vi "Digital Pattern Gen Run Test.vi"() -> ()   [LabVIEW 2013]
uses:
  IP Source/APU/Settings.ctl
  IP Source/Digital Pattern Generation/Settings.ctl
  IP Source/APU/Input.ctl
  IP Source/Digital Pattern Generation/Load Input.ctl
  <vilib>/rvi/interface/RandomDataEmulation/nirviRandomDataOpen.vi
  <vilib>/rvi/interface/common/niFpgaCacheSessionInfoDynamic.vi
  <vilib>/rvi/interface/common/niFpgaWaitOnOcc.vi
  <vilib>/Utility/error.llb/Error Cluster From Error Code.vi
  <vilib>/rvi/errors/niLvFpgaAdjustHostInterfaceError.vi
  <vilib>/FPGAPlugInAG/Dynamic/niLvFpga_Run_Dynamic.vi
  <vilib>/FPGAPlugInAG/Dynamic/niLvFpga_Close_Dynamic.vi
  <vilib>/rvi/interface/nirviOpenFPGA/nirviOpenFPGA.xnode
  Compile Tests/APU + 4 Digital Patterns.vi
  <vilib>/rvi/interface/nirviReadWriteControl/nirviReadWriteControl.xnode
  <vilib>/rvi/interface/nirviMethod/nirviMethod.xnode
  <vilib>/rvi/interface/nirviCloseFPGA/nirviCloseFPGA.xnode
  <vilib>/rvi/interface/Simulation/niFpgaSimulationCallBeginRW.vi
  IP Source/APU/APU.lvlib
  IP Source/Digital Pattern Generation/Digital Pattern Generation.lvlib
  NiFpgaLv.dll
panel:
  in  "use fault count":bool
  in  "fault count":fxp<+,4,4>
  in  "fault value":bool
  in  "fault wrap":bool
  in  "fault":bool
  in  "edge 2":u16
  in  "edge 1":u16
  in  "slow load":bool=TRUE
  in  "cycle angle":bool
  in  "Tooth Angles":cluster{"Rising Edge":dbl, "Falling Edge":dbl}[](array[cluster])=[{"Rising Edge"=50.0, "Falling Edge"=60.0}, {"Rising Edge"=100.0, "Falling Edge"=110.0}, {"Rising Edge"=200.0, "Falling Edge"=300.0}]
  out "Load done":bool
  out "Load time (s)":dbl
  in  "RPM":dbl=100000.0 format="%#_15g"
  in  "stop":bool
  # "for simulation"
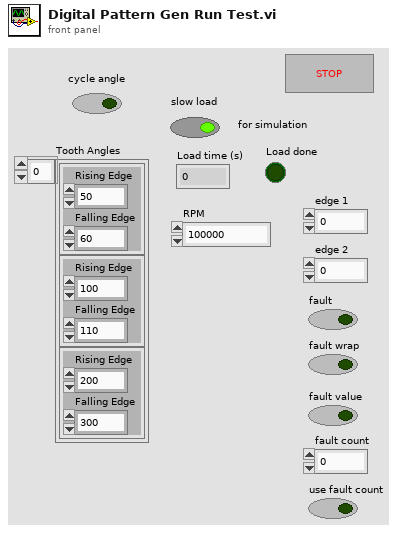
[diagram p1: front panel]
types:
  T1 = typedef "Engine Simulation Toolkit.lvlib/Digital Pattern Generation.lvlib/Settings.ctl" = cluster{"edge 1":u16, "edge 2":u16, "cycle angle":bool, "enabled":bool, "first falling":bool, "fault":bool, "fault wrap":bool, "fault value":bool, "fault count":fxp<+,4,4>, "use fault count":bool}
  T2 = typedef "Engine Simulation Toolkit.lvlib/APU.lvlib/Settings.ctl" = cluster{"acceleration":fxp<+,18,-20>, "enable accel":bool}
  T3 = typedef "Engine Simulation Toolkit.lvlib/Digital Pattern Generation.lvlib/Load Input.ctl" = cluster{"address":fxp<+,11,11>, "done":bool, "angle":u16}
  T4 = typedef "Engine Simulation Toolkit.lvlib/APU.lvlib/Input.ctl" = cluster{"desired speed":fxp<+/-,23,2>, "reset":bool}
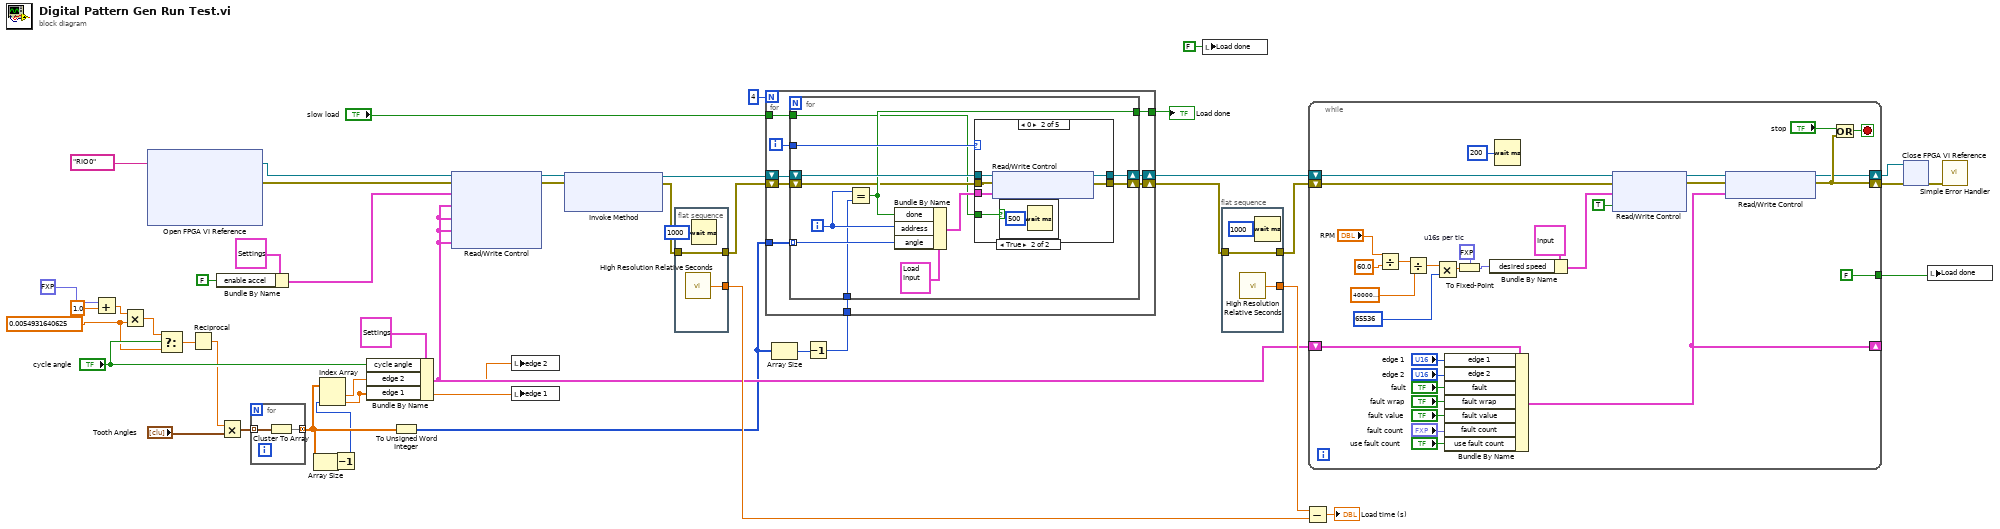
[diagram p0: block diagram]
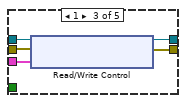
[diagram p4: hidden frame]
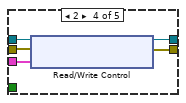
[diagram p5: hidden frame]
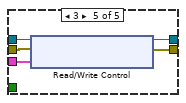
[diagram p6: hidden frame]
diagram:
  w18 = 0.0054931640625 ("x")
  n1 = Add(x=fxp<+,2,2> 1.0 ("extra cranks for a cycle"), y=1.0) -> (x+y=w6:dbl)
  n2 = Multiply(x=w6, y=w18) -> (x*y=w19:dbl)
  n3 = xnode "Open FPGA VI Reference"("resource name"=tag "RIO0") -> ("FPGA VI Reference Out"=w11:refnum<k20>, "error out"=w42:errorcluster)  [unwired: 1 in]
  n4 = Select(t=w19, s="cycle angle", f=w18) -> (s? t:f=w7:dbl)
  n5 = Reciprocal(x=w7) -> (1/x=w9:dbl)
  n6 = Bundle By Name(cluster=T2 {"acceleration"=0.0, "enable accel"=FALSE} ("settings with acceleration"), "enable accel"=FALSE) -> (w23:T2)
  n7 = Multiply(x=w9, y="Tooth Angles") -> (x*y=w16:cluster{"Rising Edge":dbl, "Falling Edge":dbl}[])
  n8 = for {
    tunnel: w16 -> [w47] mode=indexing
    tunnel: [w46] -> w14 mode=concatenating
    n9 = Cluster To Array(cluster=w47) -> (array=w46:dbl[])
  }
  n10 = Array Size(array=w14) -> (size(s)=w13:i32)
  n11 = Decrement(x=w13) -> (x-1=w12:i32)
  n12 = Index Array(array=w14, index #2=w12) -> (element #1=w1:dbl, element #2=w2:dbl)  [unwired: 1 in]
  n13 = Bundle By Name(cluster=T1 {"edge 1"=0, "edge 2"=0, "cycle angle"=TRUE, "enabled"=TRUE, "first falling"=FALSE, "fault"=FALSE, "fault wrap"=FALSE, "fault value"=FALSE, "fault count"=0.0, "use fault count"=FALSE} ("settings.<user name>"), "cycle angle"="cycle angle", "edge 2"=w1, "edge 1"=w2) -> (w10:T1)
  n14 = To Unsigned Word Integer(number=w14) -> (unsigned 16bit integer=w5:u16[])
  n15 = xnode "Read/Write Control"("FPGA VI Reference In"=w11, "error in"=w42, "settings.my apu"=w23, "settings.Pattern 1"=w10, "settings.Pattern 2"=w10, "settings.Pattern 3"=w10, "settings.Pattern 4"=w10) -> ("FPGA VI Reference Out"=w27:refnum<k20>, "error out"=w28:errorcluster)
  n16 = local write "edge 2"(w1) -> ()
  n17 = local write "edge 1"(w2) -> ()
  n18 = xnode "Invoke Method"("FPGA VI Reference In"=w27, "error in"=w28) -> ("FPGA VI Reference Out"=w38:refnum<k20>, "error out"=w36:errorcluster)  [unwired: 1 in]
  n19 = flat-sequence {
    tunnel: [w50] -> w37
    tunnel: w36 -> [w50]
    tunnel: [w49] -> w34
    frame #0 {
      n20 = call <vilib>:"High Resolution Relative Seconds.vi"() -> ("relative seconds"=w49:dbl)
      n21 = Wait (ms)(milliseconds to wait=u32 1000) -> ()  [unwired: 1 out]
    }
  }
  n22 = Array Size(array=w5) -> (size(s)=w3:i32)
  n23 = Decrement(x=w3) -> (x-1=w4:i32)
  n24 = for {
    N: 4 -> [_]
    shift-right: [w56] -> w31
    shift-left: w37 -> [w58]
    shift-right: [w57] -> w32
    shift-left: w38 -> [w59]
    tunnel: w5 -> [w55]
    tunnel: w4 -> [w53]
    tunnel: [w52] -> w15
    tunnel: "slow load" -> [w51]
    i -> [w54]
    n25 = for {
      shift-right: [w69] -> w56
      shift-left: w58 -> [w61]
      shift-right: [w70] -> w57
      shift-left: w59 -> [w71]
      tunnel: w55 -> [w67] mode=indexing
      tunnel: w54 -> [w66]
      tunnel: w53 -> [w64]
      tunnel: [w62] -> w52
      tunnel: w51 -> [w60]
      i -> [w65]
      n26 = Equal?(x=w65, y=w64) -> (x = y?=w62:bool)
      n27 = Bundle By Name(cluster=T3 {"address"=0.0, "done"=FALSE, "angle"=0} ("load input.<user name>"), "done"=w62, "address"=w65, "angle"=w67) -> (w63:T3)
      n28 = case shown="0" w66 {
        tunnel: w71 -> [w73 w79 w85 w90 w95]
        tunnel: [w73 w78 w84 w89 w94] -> w70
        tunnel: [w72 w77 w83 w88 w93] -> w69
        tunnel: w63 -> [_ w76 w82 w87 w92]
        tunnel: w61 -> [w72 w75 w81 w86 w91]
        tunnel: w60 -> [_ w74 _ _ _]
        frame Default {
        }
        frame 0 {
          n29 = xnode "Read/Write Control"("FPGA VI Reference In"=w79, "error in"=w75, "load input.Pattern 1"=w76) -> ("FPGA VI Reference Out"=w78:refnum<k20>, "error out"=w77:errorcluster)
          n30 = case shown="True" w74 {
            frame False {
            }
            frame True {
              n31 = Wait (ms)(milliseconds to wait=u32 500) -> ()  [unwired: 1 out]
            }
          }
        }
        frame 1 {
          n32 = xnode "Read/Write Control"("FPGA VI Reference In"=w85, "error in"=w81, "load input.Pattern 2"=w82) -> ("FPGA VI Reference Out"=w84:refnum<k20>, "error out"=w83:errorcluster)
        }
        frame 2 {
          n33 = xnode "Read/Write Control"("FPGA VI Reference In"=w90, "error in"=w86, "load input.Pattern 3"=w87) -> ("FPGA VI Reference Out"=w89:refnum<k20>, "error out"=w88:errorcluster)
        }
        frame 3 {
          n34 = xnode "Read/Write Control"("FPGA VI Reference In"=w95, "error in"=w91, "load input.Pattern 4"=w92) -> ("FPGA VI Reference Out"=w94:refnum<k20>, "error out"=w93:errorcluster)
        }
      }
    }
  }
  "Load done" <- w15
  n35 = local write "Load done"(FALSE ("Load done")) -> ()
  n36 = flat-sequence {
    tunnel: [w98] -> w30
    tunnel: w31 -> [w98]
    tunnel: [w97] -> w35
    frame #0 {
      n37 = call <vilib>:"High Resolution Relative Seconds.vi"() -> ("relative seconds"=w97:dbl)
      n38 = Wait (ms)(milliseconds to wait=u32 1000) -> ()  [unwired: 1 out]
    }
  }
  n39 = Subtract(x=w35, y=w34) -> (x-y=→"Load time (s)":dbl)
  n40 = while {
    shift-right: [w109] -> w45
    shift-left: w30 -> [w129]
    shift-right: [w108] -> w44
    shift-left: w32 -> [w128]
    tunnel: [FALSE ("Load")] -> w40
    shift-right: [w106] -> _
    shift-left: w10 -> [w107]
    stop <- w126 stop-if-true
    w119 = fxp<+/-,23,2> 0.0  # u16s per tic
    n41 = Divide(x="RPM", y=60.0) -> (x/y=w123:dbl)
    n42 = Divide(x=w123, y=40000000.0) -> (x/y=w120:dbl)
    n43 = Multiply(x=w120, y=u32 65536 ("n")) -> (x*y=w118:dbl)
    n44 = Bundle By Name(cluster=w107, "edge 1"="edge 1", "edge 2"="edge 2", "fault"="fault", "fault wrap"="fault wrap", "fault value"="fault value", "fault count"="fault count", "use fault count"="use fault count") -> (w106:T1)
    n45 = To Fixed-Point(fixed-point type=w119, number=w118) -> (fixed-point=w114:fxp<+/-,23,2>)
    n46 = Bundle By Name(cluster=T4 {"desired speed"=0.0, "reset"=FALSE} ("my apu"), "desired speed"=w114) -> (w113:T4)
    n47 = Wait (ms)(milliseconds to wait=u32 200) -> ()  [unwired: 1 out]
    n48 = xnode "Read/Write Control"("FPGA VI Reference In"=w128, "error in"=w129, "input.my apu"=w113, "go.my apu"=TRUE) -> ("FPGA VI Reference Out"=w110:refnum<k20>, "error out"=w111:errorcluster)
    n49 = xnode "Read/Write Control"("FPGA VI Reference In"=w110, "error in"=w111, "settings.Pattern 1"=w106) -> ("FPGA VI Reference Out"=w108:refnum<k20>, "error out"=w109:errorcluster)
    n50 = Or(x="stop", y=w109) -> (x .or. y?=w126:bool)
  }
  n51 = xnode "Close FPGA VI Reference"("FPGA VI Reference In"=w44, "error in"=w45) -> ("error out"=w43:errorcluster)
  n52 = local write "Load done"(w40) -> ()
  n53 = call <vilib>:"Simple Error Handler.vi"("error in (no error)"=w43) -> ()  [unwired: 4 in, 5 out]
